vi "Init Msg Input.vi"(6 "Teller":refnum<class "Teller.lvclass">) -> (2 "Msg Input":refnum<class "Msg Input.lvclass">)   [LabVIEW 2025, in "_Template.lvlib" / "Templates.lvlib" / "TEMPLATE jettl Msg.lvlib" / "TEMPLATE Msg Input.lvlib"]
uses:
  TEMPLATE Msg Input.lvlib
  jettl/jettl/Msg Input/Msg Input.lvclass
  jettl/jettl/Teller/Teller.lvclass
  TEMPLATE Msg Input/TEMPLATE Msg Input.lvclass
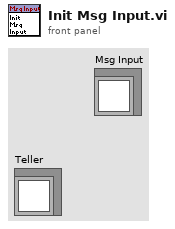
[diagram p1: front panel]
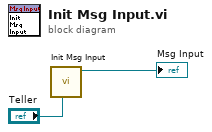
[diagram p0: block diagram]
diagram:
  n1 = call "Init Msg Input.vi"("Teller"="Teller") -> ("TEMPLATE Msg Input out"=→"Msg Input":refnum<class "TEMPLATE Msg Input.lvclass">)  [unwired: 10 in]
